vi "NIFPGA-MCS.get library version.vi"() -> (0 "nameAndVersion":string)   [LabVIEW 2014, in "NIFPGA-MCS.lvlib"]
doc: "obtain name and version of a library as a string"
uses:
  NIFPGA-MCS.lvlib
  CSlibraries/UtilityLib/UtilityLib.lvlib
  CSinstr.lib/NI-FPGA-MCS/host/instrumentDriver/NI-FPGA-MCS_Driver.lvlib
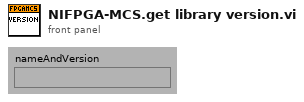
[diagram p1: front panel]
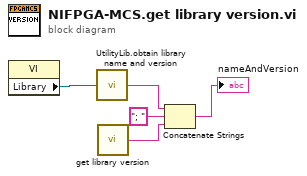
[diagram p0: block diagram]
diagram:
  n1 = property class="VI"() -> ("Library"=w5:refnum<vi>)  [unwired: 2 in, 2 out]
  n2 = call "UtilityLib.obtain library name and version.vi"("Library"=w5) -> ("nameAndVersion"=w3:string)
  n3 = call "get library version.vi"() -> ("nameAndVersion"=w2:string)  [unwired: 1 in]
  n4 = Concatenate Strings(w3, "; " ("string"), w2) -> (→"nameAndVersion":string)
